vi "Panel Initialize.vi"(8 "error in":errorcluster, 10 "Initialize All UI ?":bool, 11 "VI Ref":refnum<vi>) -> (0 "error out":errorcluster, 1 "Ver.#":string, 3 "Structure Data":T1)   [LabVIEW 2020]
uses:
  Def/Main_Data_Package.ctl
  Def/Queue_Method Def.ctl
  Def/User_Event.ctl
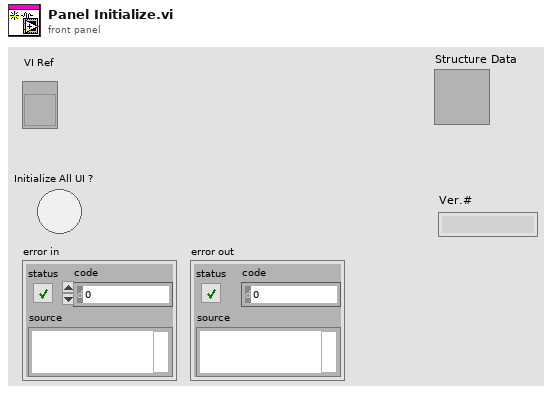
[diagram p1: front panel]
types:
  T1 = typedef "Main_Data_Package.ctl" = cluster{"This Vi Ref Out":refnum<vi>, "Map Out":map{string, refnum<vi>}, "User Event Out":refnum<user-event>, "User_Event Ref Reg":refnum<event-registration>, "Event Log Path":path}
  T2 = typedef "Queue_Method Def.ctl" = enum16{"Initialize", "Read", "Write", "Insert", "Get_Specific_Quene_Status", "Flush Speciffic Quene", "Release All Quenes"}
  T3 = enum16{"Initialize", "Get", "Read", "Write", "Release"}
  T4 = typedef "User_Event.ctl" = cluster{"String":string, "Data":variant}
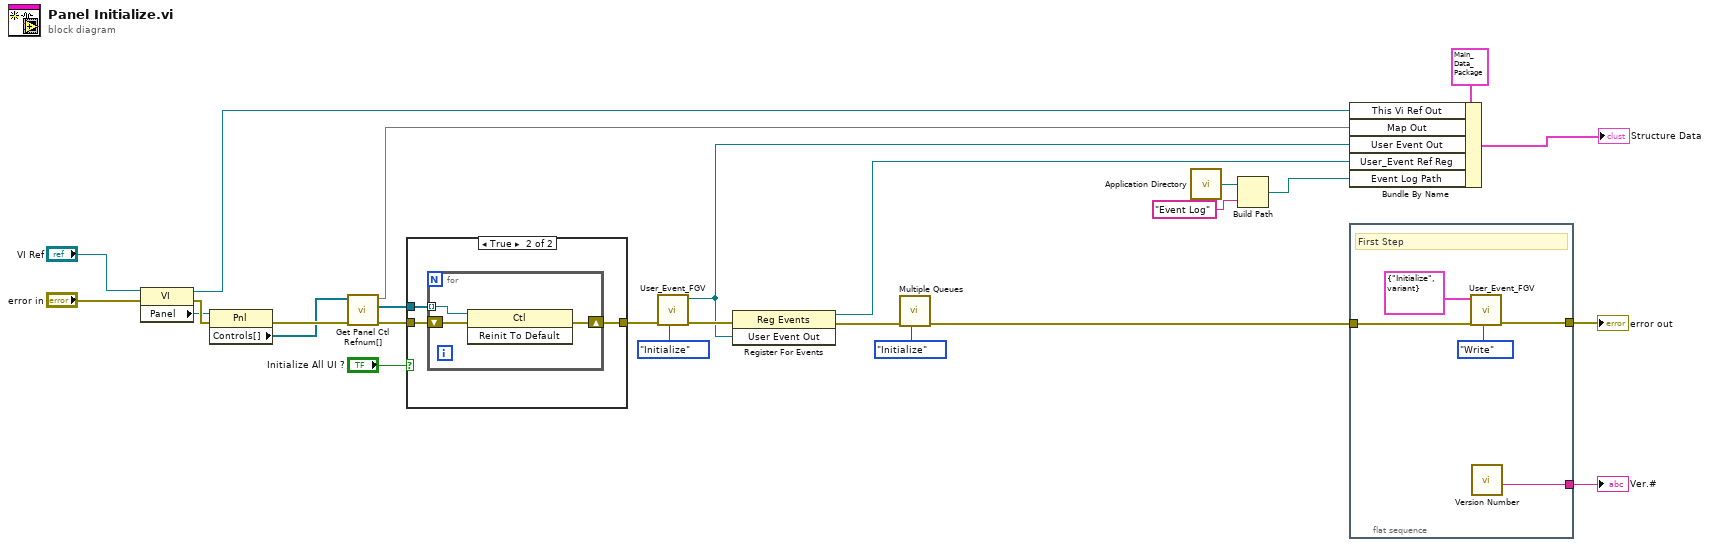
[diagram p0: block diagram]
diagram:
  n1 = property on="Property Node" class="VI"(reference="VI Ref", error in="error in") -> (reference out=w9:refnum<vi>, error out=w26:errorcluster, "Panel"=w25:refnum<vi>)
  n2 = property on="Property Node" class="Pnl"(reference=w25, error in=w26) -> (error out=w21:errorcluster, "Controls[]"=w16:refnum<vi>[])  [unwired: 1 out]
  n3 = call "Get Panel Ctl Refnum[].vi"("error in"=w21, "Controls[]"=w16) -> ("error out"=w20:errorcluster, "Controls[] Out"=w17:refnum<vi>[], "Map Out"=w8:map{string, refnum<vi>})  [unwired: 7 in]
  n4 = case shown="True" "Initialize All UI ?" {
    tunnel: [w27 w30] -> w19
    tunnel: w20 -> [w27 w29]
    tunnel: w17 -> [_ w28]
    frame False {
    }
    frame True {
      n5 = for {
        shift-right: [w32] -> w30
        shift-left: w29 -> [w33]
        tunnel: w28 -> [w31] mode=indexing
        n6 = invoke class="Ctl" method="Reinit To Default"(reference=w31, error in=w33) -> (error out=w32:errorcluster)  [unwired: 1 in, 2 out]
      }
    }
  }
  n7 = call "User_Event_FGV.vi"("Method"=T3."Initialize", "error in"=w19) -> ("error out"=w12:errorcluster, "User Event Out"=w4:refnum<user-event>)  [unwired: 8 in]
  n8 = register-events(error in=w12, w4) -> (reference out=w7:refnum<event-registration>, error out=w11:errorcluster)  [unwired: 1 in]
  n9 = call "Multiple Queues.vi"("Method"=Queue_Method_Def."Initialize", "error in"=w11) -> ("error out"=w6:errorcluster)  [unwired: 7 in, 2 out]
  n10 = call <vilib>:"Application Directory.vi"() -> ("Application Directory"=w3:path)
  n11 = Build Path(base path=w3, name or relative path="Event Log") -> (appended path=w2:path)
  n12 = Bundle By Name(cluster=T1 {"This Vi Ref Out"=refnum, "Map Out"={}, "User Event Out"=refnum, "User_Event Ref Reg"=refnum, "Event Log Path"=path ""} ("Cluster"), "This Vi Ref Out"=w9, "Map Out"=w8, "User Event Out"=w4, "User_Event Ref Reg"=w7, "Event Log Path"=w2) -> (→"Structure Data":T1)
  n13 = flat-sequence {
    tunnel: [w37] -> w15
    tunnel: [w35] -> w14
    tunnel: w6 -> [w34]
    frame #0 {
      # "First Step"
      n14 = call "User_Event_FGV.vi"("Method"=T3."Write", "error in"=w34, "User Event"=T4 {"String"="Initialize", "Data"=variant}) -> ("error out"=w37:errorcluster)  [unwired: 7 in, 1 out]
      n15 = call "Version Number.vi"() -> ("Version Number"=w35:string)  [unwired: 11 in]
    }
  }
  "error out" <- w15
  "Ver.#" <- w14
